vi "Update VF Device.vi"(10 "IED_Status":variant, 11 "EMS in":refnum<class "EMS.lvclass">) -> ()   [LabVIEW 2018, in "EMS Core.lvlib" / "EMS.lvclass"]
uses:
  EMS.lvclass
  C:/Users/Administrator/Desktop/LabVIEW EMS/EMS Generic Actor/EMS Generic/EMS Generic.lvclass
  EMS Generic Actor/EMS Generic/EMS Generic.lvclass/EMS Generic.ctl
  EMS Generic Actor/EMS Generic/Accessors - Global Configuration/Read Global Configuration.vi
  EMS Generic Actor/EMS Generic/Accessors - Global Configuration/Update Global Configuration.vi
  EMS Generic Actor/EMS Generic/EMS Generic.lvclass
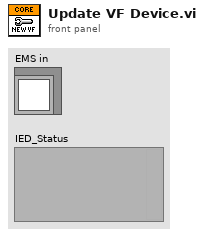
[diagram p1: front panel]
types:
  T1 = typedef "CSEISMIC DDS.lvlib/CSEISMIC DDS.lvclass/DeviceID.ctl" = string
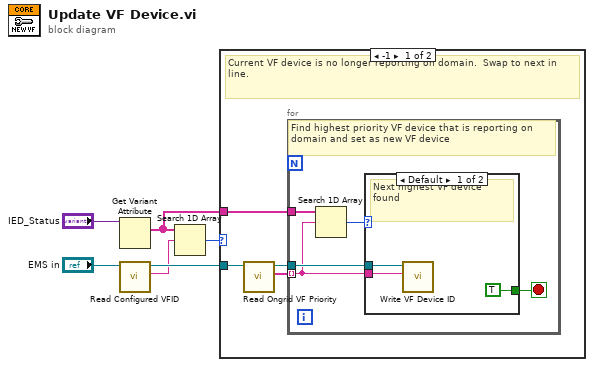
[diagram p0: block diagram]
diagram:
  n1 = Get Variant Attribute(Variant="IED_Status") -> (names=w1:string[])  [unwired: 3 in, 3 out]
  n2 = call "Read Configured VFID.vi"("EMS Generic in"="EMS in") -> ("VFID"=w3:T1, "EMS Generic out"=w4:refnum<class "EMS.lvclass">)  [unwired: 8 in, 1 out]
  n3 = Search 1D Array(1D array=w1, element=w3) -> (index of element=w2:i32)  [unwired: 1 in]
  n4 = case shown="-1" w2 {
    tunnel: w4 -> [w10 _]
    tunnel: w1 -> [w8 _]
    frame -1 {
      # "Current VF device is no longer reporting on domain.  Swap to next in line."
      n5 = call "Read Ongrid VF Priority.vi"("EMS Generic in"=w10) -> ("Ongrid VF Priority"=w9:T1[], "EMS Generic out"=w7:refnum<class "EMS.lvclass">)  [unwired: 8 in, 1 out]
      n6 = for {
        tunnel: w9 -> [w12] mode=indexing
        tunnel: w8 -> [w15]
        tunnel: w7 -> [w13]
        stop <- w11 stop-if-true
        # "Find highest priority VF device that is reporting on domain and set as new VF device"
        n7 = Search 1D Array(1D array=w15, element=w12) -> (index of element=w14:i32)  [unwired: 1 in]
        n8 = case shown="Default" w14 {
          tunnel: w13 -> [w18 _]
          tunnel: w12 -> [w17 _]
          tunnel: [TRUE _] -> w11
          frame Default {
            # "Next highest VF device found"
            n9 = call "Write VF Device ID.vi"("VF Device"=w17, "EMS Generic in"=w18) -> ()  [unwired: 8 in, 2 out]
          }
          frame -1 {
            # "Backup VF device not reporting on domain"
          }
        }
      }
    }
    frame Default {
      # "Current VF device is still reporting on the domain.  Do nothing."
    }
  }
